vi "Close Front Panel.vi"(8 "error in":errorcluster, 11 "VI Reference":refnum<vi>) -> (0 "error out":errorcluster)   [LabVIEW 2022 SP3]
doc: "Closes the Front Panel, but only when the VI is called from within the Shortcut Menu framework, not when the VI is run in development environment for development and testing."
uses:
  Testing Flag (library variable).vi
panel:
  # "Development\ncontrols/indicators useful for development and testing, but which are not outputs of the VI"
  # "Input\nInputs to the VI"
  # "Output\nOutputs of the VI"
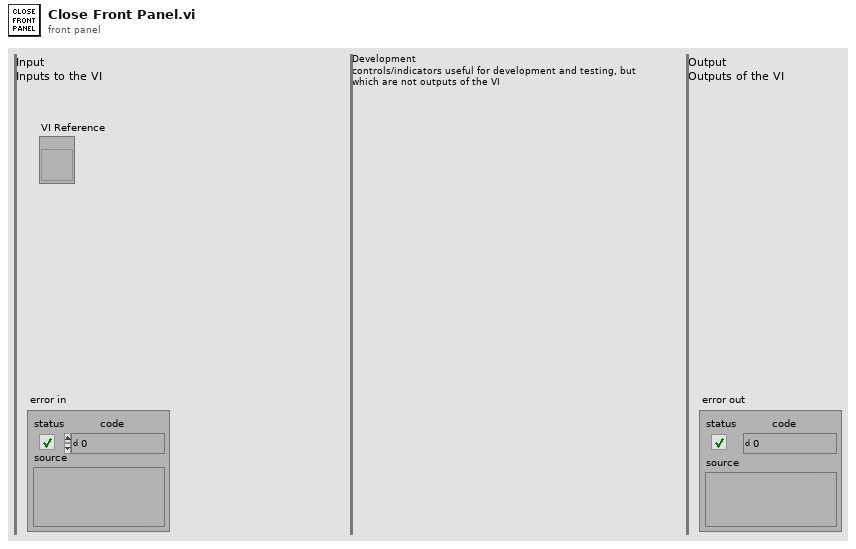
[diagram p1: front panel]
types:
  T1 = typedef "Testing Flag (enum).ctl" = enum16{"Production", "Testing"}
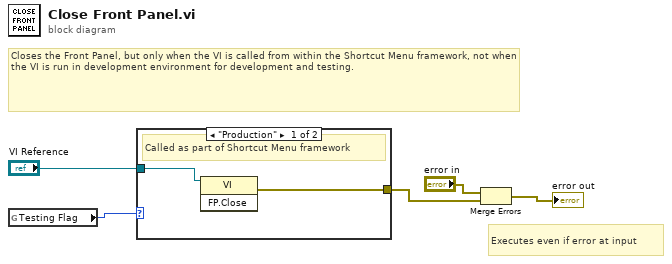
[diagram p0: block diagram]
diagram:
  # "Executes even if error at input"
  # "Closes the Front Panel, but only when the VI is called from within the Shortcut Menu framework, not when the VI is run in development environment for development and testing."
  n1 = global read "Testing Flag (library variable).vi" "Testing Flag"() -> (w1:T1)
  n2 = case shown="\"Production\"" w1 {
    tunnel: "VI Reference" -> [w7 _]
    tunnel: [w6 _] -> w4
    frame "Production" {
      # "Called as part of Shortcut Menu framework"
      n3 = invoke class="VI" method="FP.Close"(reference=w7) -> (error out=w6:errorcluster)  [unwired: 2 in, 2 out]
    }
    frame "Testing" {
      # "Called from dev environment (during dev and test)"
    }
  }
  n4 = Merge Errors("error in", w4) -> (→"error out":errorcluster)
